vi "final_project.vi"() -> ()   [LabVIEW 2020]
panel:
  out "moisture":dbl(knob) scale=0.0..100.0
  out "ph":dbl(knob) scale=0.0..14.0
  out "ph Chart":dbl(graph)
  in  "VISA resource name":refnum<visa-resource-name>
  in  "Table Control":string[][](table)
  out "humidity Chart":dbl(graph)
  out "temp Chart":dbl(graph)
  out "Humidity":dbl(knob) scale=0.0..100.0
  out "Temp":dbl(slide) scale=0.0..100.0
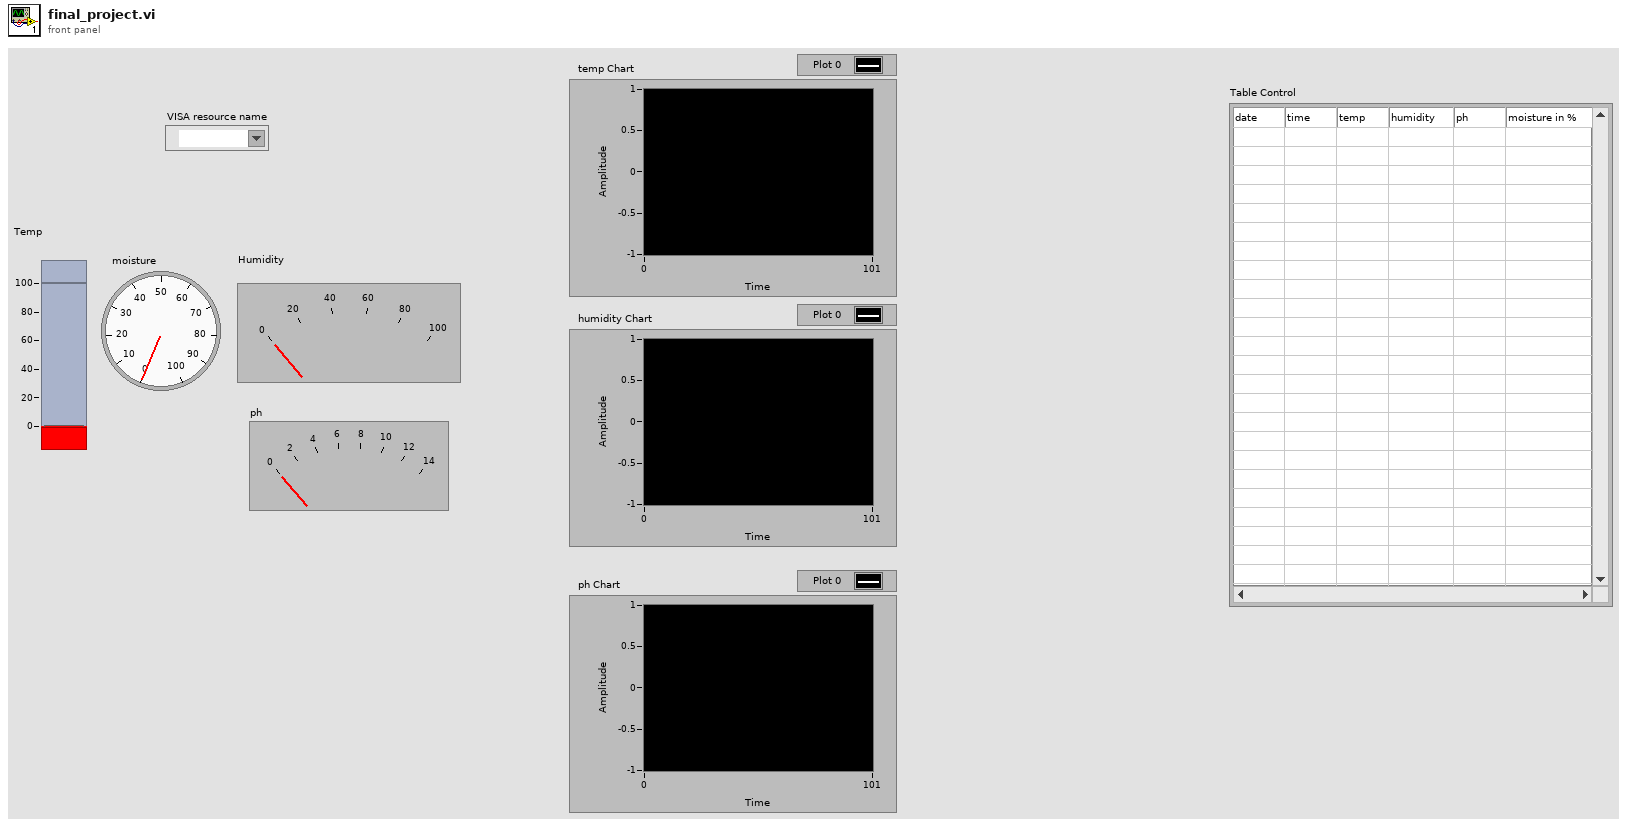
[diagram p1: front panel]
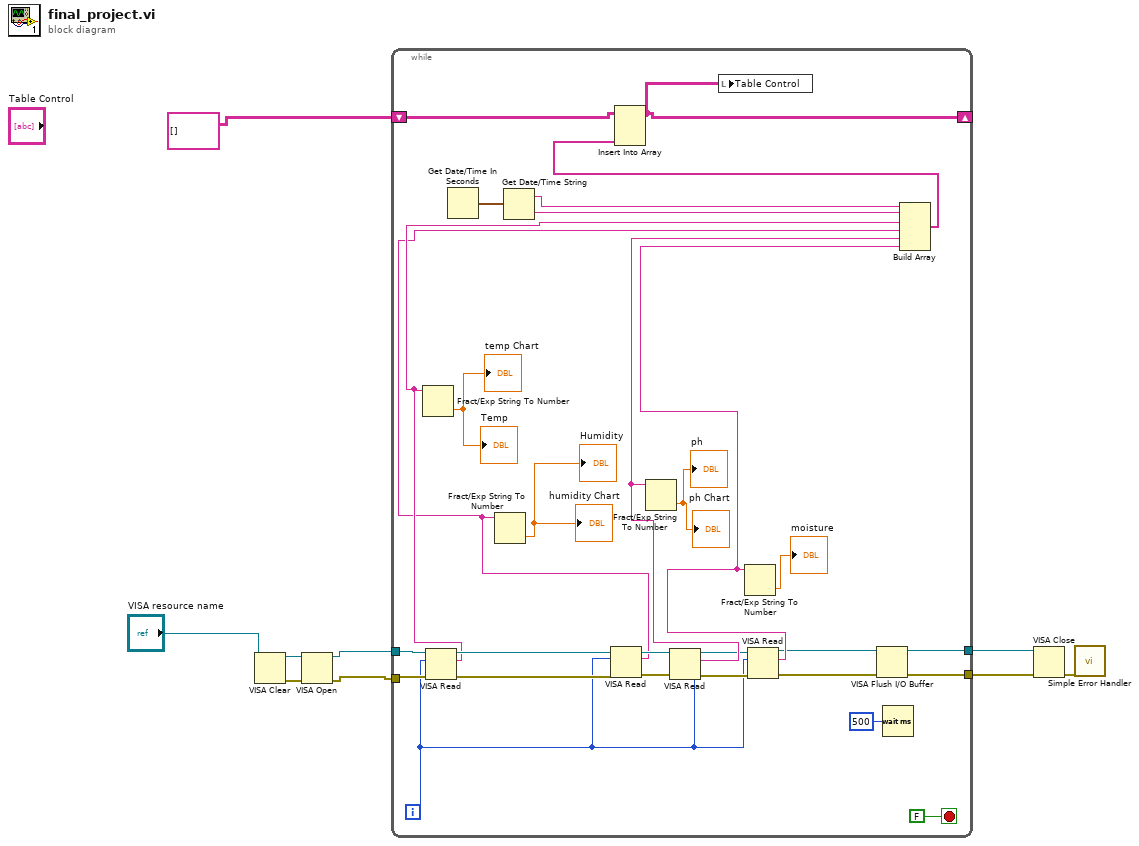
[diagram p0: block diagram]
diagram:
  n1 = VISA Clear(VISA resource name="VISA resource name") -> (VISA resource name out=w8:refnum<visa-resource-name>, error out=w7:errorcluster)  [unwired: 1 in]
  n2 = VISA Open(error in (no error)=w7, VISA resource name=w8) -> (VISA resource name=w6:refnum<visa-resource-name>, error out=w5:errorcluster)  [unwired: 3 in]
  n3 = while {
    tunnel: w6 -> [w38]
    tunnel: w5 -> [w37]
    tunnel: [w34] -> w4
    tunnel: [w33] -> w3
    shift-right: [w17] -> _
    shift-left: string[][] [] -> [w19]
    i -> [w14]
    stop <- FALSE stop-if-true
    n4 = VISA Read(VISA resource name=w38, byte count=w14, error in (no error)=w37) -> (VISA resource name out=w35:refnum<visa-resource-name>, read buffer=w23:string, error out=w36:errorcluster)  [unwired: 1 out]
    n5 = Fract/Exp String To Number(string=w23) -> (number=→"Temp" →"temp Chart":dbl)  [unwired: 3 in, 1 out]
    n6 = Get Date/Time In Seconds() -> (seconds since 1Jan1904=w29:timestamp)
    n7 = Get Date/Time String(seconds (now)=w29) -> (date string=w28:string, time string=w27:string)  [unwired: 2 in]
    n8 = VISA Read(VISA resource name=w35, byte count=w14, error in (no error)=w36) -> (VISA resource name out=w25:refnum<visa-resource-name>, read buffer=w22:string, error out=w24:errorcluster)  [unwired: 1 out]
    n9 = Fract/Exp String To Number(string=w22) -> (number=→"Humidity" →"humidity Chart":dbl)  [unwired: 3 in, 1 out]
    n10 = VISA Read(VISA resource name=w25, byte count=w14, error in (no error)=w24) -> (VISA resource name out=w16:refnum<visa-resource-name>, read buffer=w20:string, error out=w15:errorcluster)  [unwired: 1 out]
    n11 = Fract/Exp String To Number(string=w20) -> (number=→"ph Chart" →"ph":dbl)  [unwired: 3 in, 1 out]
    n12 = VISA Read(VISA resource name=w16, byte count=w14, error in (no error)=w15) -> (VISA resource name out=w11:refnum<visa-resource-name>, read buffer=w13:string, error out=w10:errorcluster)  [unwired: 1 out]
    n13 = Fract/Exp String To Number(string=w13) -> (number=→"moisture":dbl)  [unwired: 3 in, 1 out]
    n14 = VISA Flush I/O Buffer(VISA resource name=w11, error in (no error)=w10) -> (VISA resource name out=w34:refnum<visa-resource-name>, error out=w33:errorcluster)  [unwired: 1 in]
    n15 = Wait (ms)(milliseconds to wait=u32 500) -> ()  [unwired: 1 out]
    n16 = Build Array(w28, w27, w23, w22, w20, w13) -> (w18:string[])
    n17 = Insert Into Array(array=w19, new element=w18) -> (w17:string[][])  [unwired: 2 in]
    n18 = local write "Table Control"(w17) -> ()
  }
  n19 = VISA Close(VISA resource name=w4, error in (no error)=w3) -> (error out=w9:errorcluster)
  n20 = call <vilib>:"Simple Error Handler.vi"("error in (no error)"=w9) -> ()  [unwired: 4 in, 5 out]
